vi "DeleteRow.vi"(8 "error":errorcluster caption="错误输入（无错误）", 9 "Second":string, 10 "First":string, 11 "Excel._Worksheet":refnum<k7>) -> (0 "error out":errorcluster caption="错误输出", 3 "Excel._Worksheet":refnum<k7>)   [LabVIEW 2014]
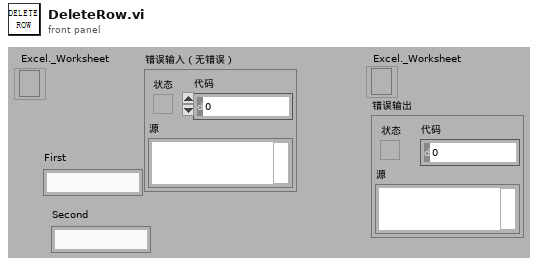
[diagram p1: front panel]
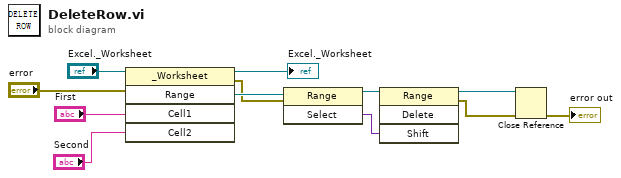
[diagram p0: block diagram]
diagram:
  n1 = invoke class="_Worksheet" method="Range"(reference="Excel._Worksheet", error in="error", "Cell1"="First", "Cell2"="Second") -> (reference out=→"Excel._Worksheet":refnum<k7>, error out=w2:errorcluster, "Range"=w7:refnum<k7>)  [unwired: 1 in, 2 out]
  n2 = invoke class="Range" method="Select"(reference=w7, error in=w2) -> (reference out=w6:refnum<k7>, "Select"=w5:variant)  [unwired: 1 in, 1 out]
  n3 = invoke class="Range" method="Delete"(reference=w6, "Shift"=w5) -> (reference out=w4:refnum<k7>, error out=w3:errorcluster)  [unwired: 2 in, 2 out]
  n4 = Close Reference(reference=w4, error in (no error)=w3) -> (error out=→"error out":errorcluster)
